vi "FilterBasedIntegration.vi"(8 "error in (no error)":errorcluster, 10 "Integration Properties in":T1={"Conversion Op"=enum."singleInt", "Unit"="", "Parent Unit"="", "Single Integration Cutoff"=0.0, "Double Integration Cutoff"=0.0, "Lowpass Filter State"={"designed"=FALSE, "integration filter coefficients"={"beta"=0.0, "gamma"=0.0, "alpha"=0.0}, "state"={"x(n-1) state"=0.0, "y(n-1) state"=0.0, "x(n-2) state"=0.0, "y(n-2) state"=0.0}}, "Highpass Filter State"={"designed"=FALSE, "IIR Filter Cluster"={"filter structure"=enum."IIR 2nd Order", "Reverse Coefficients"=[], "Forward Coefficients"=[]}, "Filter State"=[]}, "Wfm Scale"=0.0} {"Highpass Filter State"."Filter State" format="%.2f"; "Highpass Filter State"."IIR Filter Cluster"."Forward Coefficients" format="%.2f"; "Highpass Filter State"."IIR Filter Cluster"."Reverse Coefficients" format="%.2f"; "Lowpass Filter State"."state"."y(n-2) state" format="%.2f"; "Lowpass Filter State"."state"."x(n-2) state" format="%.2f"; "Lowpass Filter State"."state"."y(n-1) state" format="%.2f"; "Lowpass Filter State"."state"."x(n-1) state" format="%.2f"}, 11 "Waveform":waveform(sgl)={"t0"=timestamp(0 s since 1904-01-01), "dt"=0.0, "Y"=[]}) -> (0 "error out":errorcluster, 2 "Integration Properties out":T1={"Conversion Op"=enum."singleInt", "Unit"="", "Parent Unit"="", "Single Integration Cutoff"=0.0, "Double Integration Cutoff"=0.0, "Lowpass Filter State"={"designed"=FALSE, "integration filter coefficients"={"beta"=0.0, "gamma"=0.0, "alpha"=0.0}, "state"={"x(n-1) state"=0.0, "y(n-1) state"=0.0, "x(n-2) state"=0.0, "y(n-2) state"=0.0}}, "Highpass Filter State"={"designed"=FALSE, "IIR Filter Cluster"={"filter structure"=enum."IIR 2nd Order", "Reverse Coefficients"=[], "Forward Coefficients"=[]}, "Filter State"=[]}, "Wfm Scale"=0.0} {"Highpass Filter State"."Filter State" format="%.2f"; "Highpass Filter State"."IIR Filter Cluster"."Forward Coefficients" format="%.2f"; "Highpass Filter State"."IIR Filter Cluster"."Reverse Coefficients" format="%.2f"; "Lowpass Filter State"."state"."y(n-2) state" format="%.2f"; "Lowpass Filter State"."state"."x(n-2) state" format="%.2f"; "Lowpass Filter State"."state"."y(n-1) state" format="%.2f"; "Lowpass Filter State"."state"."x(n-1) state" format="%.2f"}, 3 "Integrated Waveform":waveform(sgl))   [LabVIEW 2017, in "CmsVirtualChannel.lvlib"]
uses:
  <vilib>/addons/InsightCM/Devices/Shared/Cms/CmsVirtualChannel/CmsVirtualChannel.lvlib
  <vilib>/addons/InsightCM/Devices/Shared/Cms/CmsVirtualChannel/controls/Integration.ctl
  <vilib>/addons/InsightCM/Utilities/Analysis/Shared/controls/ConversionOp.ctl
  <vilib>/addons/InsightCM/Utilities/Analysis/Vibration/controls/LowPassFilterState.ctl
  <vilib>/addons/InsightCM/Utilities/Analysis/Vibration/controls/HighPassFilterState.ctl
  <vilib>/addons/InsightCM/Utilities/Analysis/Vibration/VibrationAnalysisFunctions.lvlib
  <vilib>/addons/InsightCM/Utilities/Analysis/Shared/AnalysisHelper.lvlib
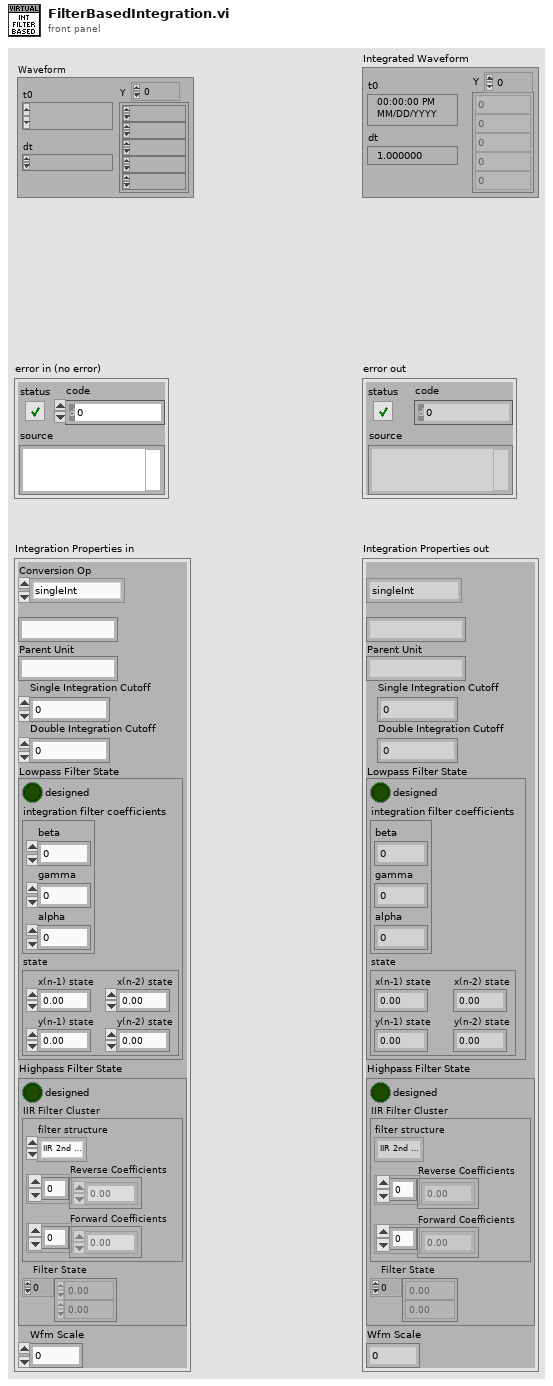
[diagram p1: front panel]
types:
  T1 = typedef "CmsVirtualChannel.lvlib/Integration.ctl" = cluster{"Conversion Op":T2, "Unit":string, "Parent Unit":string, "Single Integration Cutoff":dbl, "Double Integration Cutoff":dbl, "Lowpass Filter State":T3, "Highpass Filter State":T4, "Wfm Scale":sgl}
  T2 = typedef "AnalysisHelper.lvlib/ConversionOp.ctl" = enum16{"none", "singleInt", "doubleInt", "singleDiff", "doubleDiff"}
  T3 = typedef "VibrationAnalysisFunctions.lvlib/LowPassFilterState.ctl" = cluster{"designed":bool, "integration filter coefficients":cluster{"beta":dbl, "gamma":dbl, "alpha":dbl}, "state":cluster{"x(n-1) state":dbl, "y(n-1) state":dbl, "x(n-2) state":dbl, "y(n-2) state":dbl}}
  T4 = typedef "VibrationAnalysisFunctions.lvlib/HighPassFilterState.ctl" = cluster{"designed":bool, "IIR Filter Cluster":cluster{"filter structure":enum32{"IIR 2nd Order", "IIR 4th Order"}, "Reverse Coefficients":dbl[], "Forward Coefficients":dbl[]}, "Filter State":dbl[]}
  T5 = cluster{"x(n-1) state":dbl, "y(n-1) state":dbl, "x(n-2) state":dbl, "y(n-2) state":dbl}
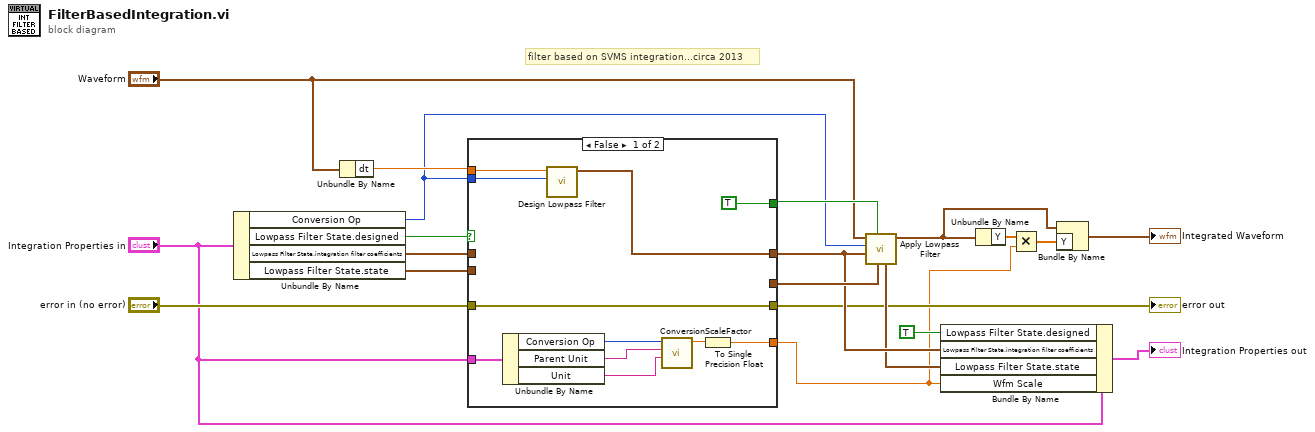
[diagram p0: block diagram]
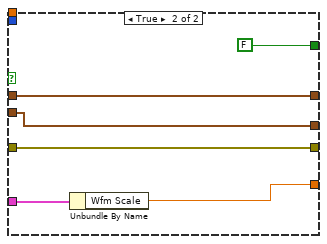
[diagram p2: hidden frame]
diagram:
  # "filter based on SVMS integration...circa 2013"
  n1 = Unbundle By Name("Integration Properties in") -> ("Conversion Op"=w5:T2, "Lowpass Filter State.designed"=w16:bool, "Lowpass Filter State.integration filter coefficients"=w15:cluster{"beta":dbl, "gamma":dbl, "alpha":dbl}, "Lowpass Filter State.state"=w14:T5)
  n2 = Unbundle By Name("Waveform") -> ("dt"=w6:dbl)
  n3 = case shown="False" w16 {
    tunnel: "error in (no error)" -> [w31 w37]
    tunnel: [w31 w37] -> w9
    tunnel: [w29 w35] -> w12
    tunnel: [_ w34] -> w19
    tunnel: [TRUE FALSE] -> w18
    tunnel: w5 -> [w28 _]
    tunnel: w15 -> [_ w35]
    tunnel: w14 -> [_ w34]
    tunnel: w6 -> [w27 _]
    tunnel: "Integration Properties in" -> [w23 w33]
    tunnel: [w21 w32] -> w1
    frame False {
      n4 = Unbundle By Name(w23) -> ("Conversion Op"=w24:T2, "Parent Unit"=w25:string, "Unit"=w26:string)
      n5 = call <vilib>:"Design Lowpass Filter.vi"("Conversion Op"=w28, "dt"=w27) -> ("filter coefficients"=w29:cluster{"beta":dbl, "gamma":dbl, "alpha":dbl})  [unwired: 9 in]
      n6 = call <vilib>:"ConversionScaleFactor.vi"("Desired Unit"=w26, "Original Unit"=w25, "Conversion Op"=w24) -> ("Scale Factor"=w22:dbl)  [unwired: 8 in]
      n7 = To Single Precision Float(number=w22) -> (single precision float=w21:sgl)
    }
    frame True {
      n8 = Unbundle By Name(w33) -> ("Wfm Scale"=w32:sgl)
    }
  }
  "error out" <- w9
  n9 = call <vilib>:"Apply Lowpass Filter.vi"("state info in"=w19, "reset"=w18, "filter coefficients"=w12, "Conversion Op"=w5, "Input stream"="Waveform") -> ("filtered signal"=w17:waveform(sgl), "state info out"=w11:T5)  [unwired: 5 in]
  n10 = Bundle By Name(cluster="Integration Properties in", "Lowpass Filter State.designed"=TRUE ("designed"), "Lowpass Filter State.integration filter coefficients"=w12, "Lowpass Filter State.state"=w11, "Wfm Scale"=w1) -> (→"Integration Properties out":T1)
  n11 = Unbundle By Name(w17) -> ("Y"=w4:sgl[])
  n12 = Multiply(x=w4, y=w1) -> (x*y=w3:sgl[])
  n13 = Bundle By Name(cluster=w17, "Y"=w3) -> (→"Integrated Waveform":waveform(sgl))
